vi "CMD SetAcqMode.vi"(8 "error in (no error)":errorcluster, 10 "Acqusition Mode":T1, 11 "DAQ_Engine in":refnum<class "DAQ_Engine.lvclass">) -> (0 "error out":errorcluster, 3 "DAQ_Engine out":refnum<class "DAQ_Engine.lvclass">)   [LabVIEW 2019, in "DAQ_Engine.lvclass"]
doc: "Developed by Kevin Thompson\nkevin@thompsonengineering.net\n\nCopyright 2018\nThompson Engineering, LLC"
uses:
  DAQ_Engine.lvclass
  DataTypes/AsynCmd_DAQ_Engine--enum.ctl
  Common/DataTypes/Acquisition Mode--cluster.ctl
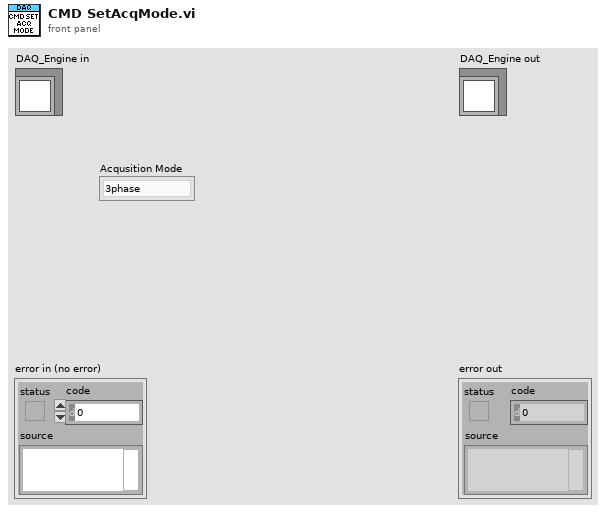
[diagram p1: front panel]
types:
  T1 = typedef "Acquisition Mode--cluster.ctl" = enum16{"3phase", "Single"}
  T2 = typedef "DAQ_Engine.lvclass/AsynCmd_DAQ_Engine--enum.ctl" = enum16{"DAQ.EnableDAQ", "DAQ.ClearDAQError", "DAQ.SetMeasConfig", "DAQ.SetAcqMode", "DAQ.SetErrorReporting"}
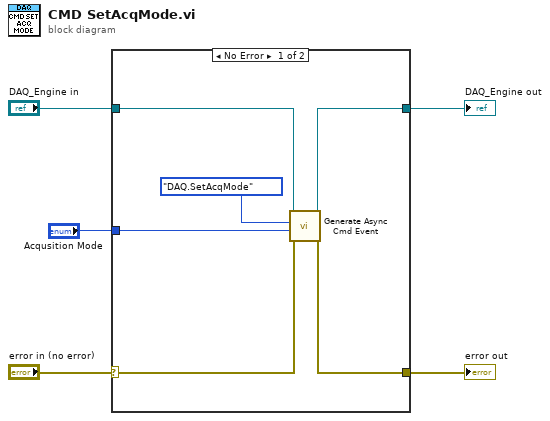
[diagram p0: block diagram]
diagram:
  n1 = case shown="No Error" "error in (no error)" {
    selector: "error in (no error)" -> [w9 w13]
    tunnel: [w8 w13] -> w4
    tunnel: [w10 w12] -> w2
    tunnel: "DAQ_Engine in" -> [w11 w12]
    tunnel: "Acqusition Mode" -> [w6 _]
    frame No Error {
      n2 = call "Generate Async Cmd Event.vi"("error in (no error)"=w9, "vData"=w6, "AsyncCmd"=AsynCmd_DAQ_Engine--enum."DAQ.SetAcqMode", "DAQ_Engine in"=w11) -> ("error out"=w8:errorcluster, "DAQ_Engine out"=w10:refnum<class "DAQ_Engine.lvclass">)  [unwired: 6 in]
    }
    frame Error {
    }
  }
  "error out" <- w4
  "DAQ_Engine out" <- w2
